vi "Ex6.vi"() -> ()   [LabVIEW 2016]
uses:
  <vilib>/DAQmx/create/channels.llb/DAQmx Create Channel (CO-Pulse Generation-Frequency).vi
  <vilib>/DAQmx/configure/timing.llb/DAQmx Timing (Implicit).vi
  <vilib>/DAQmx/miscellaneous.llb/DAQmx Fill In Error Info.vi
  <vilib>/DAQmx/create/channels.llb/DAQmx Create Channel (CI-Period).vi
  <vilib>/DAQmx/read.llb/DAQmx Read (Counter DBL 1Chan 1Samp).vi
panel:
  in  "frequency":dbl=1.0 caption="주파수" format="%.6f"
  in  "counter 2":tag caption="카운터"
  out "data":dbl caption="주기" format="%.8p"
  in  "counter":tag caption="카운터"
  in  "정지":bool
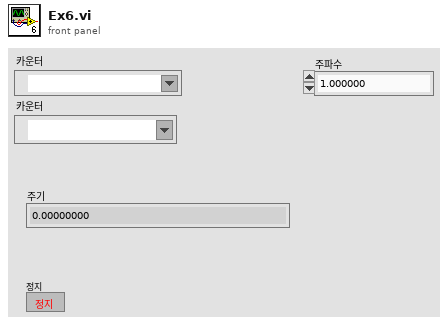
[diagram p1: front panel]
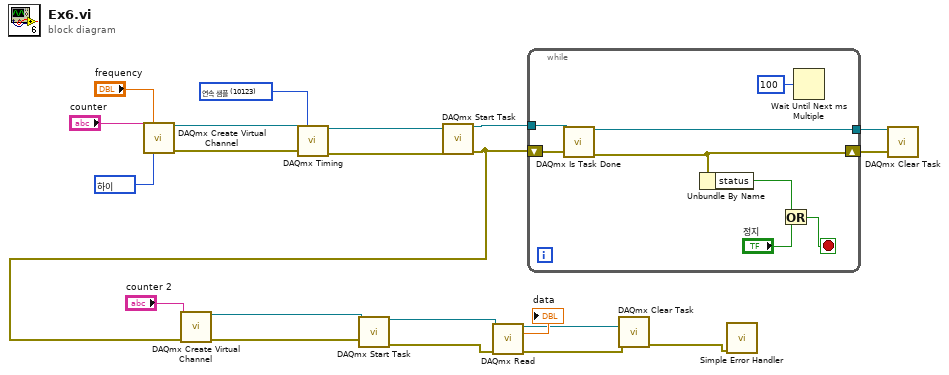
[diagram p0: block diagram]
diagram:
  w1 = 10192 items=["하이"=10192, "로우"=10214] ("idle state")
  w13 = 10123 items=["유한 샘플"=10178, "연속 샘플"=10123, "하드웨어 타이밍에 의한 단일 포인트"=12522] ("sample mode")
  n1 = call-poly <vilib>:"DAQmx Create Virtual Channel.vi"("frequency"="frequency", "counter"="counter", "idle state"=w1) -> ("task out"=w21:refnum<k21>, "error out"=w20:errorcluster)  [unwired: 11 in]
  n2 = call-poly <vilib>:"DAQmx Timing.vi"("task/channels in"=w21, "sample mode"=w13, "error in"=w20) -> ("task out"=w16:refnum<k21>, "error out"=w15:errorcluster)  [unwired: 11 in]
  n3 = call <vilib>:"DAQmx Start Task.vi"("task/channels in"=w16, "error in"=w15) -> ("task out"=w14:refnum<k21>, "error out"=w4:errorcluster)  [unwired: 12 in]
  n4 = call-poly <vilib>:"DAQmx Create Virtual Channel.vi"("counter"="counter 2", "error in"=w4) -> ("task out"=w12:refnum<k21>, "error out"=w11:errorcluster)  [unwired: 12 in]
  n5 = call <vilib>:"DAQmx Start Task.vi"("task/channels in"=w12, "error in"=w11) -> ("task out"=w10:refnum<k21>, "error out"=w9:errorcluster)  [unwired: 12 in]
  n6 = call-poly <vilib>:"DAQmx Read.vi"("task/channels in"=w10, "error in"=w9) -> ("task out"=w7:refnum<k21>, "data"=→"data":dbl, "error out"=w6:errorcluster)  [unwired: 11 in]
  n7 = while {
    shift-right: [w27] -> w19
    shift-left: w4 -> [w29]
    tunnel: [w28] -> w18
    tunnel: w14 -> [w23]
    stop <- w24 stop-if-true
    n8 = call <vilib>:"DAQmx Is Task Done.vi"("task/channels in"=w23, "error in"=w29) -> ("task out"=w28:refnum<k21>, "error out"=w27:errorcluster)  [unwired: 11 in, 1 out]
    n9 = Unbundle By Name(w27) -> ("status"=w26:bool)
    n10 = Or(x=w26, y="정지") -> (x .or. y?=w24:bool)
    n11 = Wait Until Next ms Multiple(millisecond multiple=u32 100 ("대기 시간 (ms)")) -> ()  [unwired: 1 out]
  }
  n12 = call <vilib>:"DAQmx Clear Task.vi"("task in"=w7, "error in"=w6) -> ("error out"=w5:errorcluster)  [unwired: 13 in]
  n13 = call <vilib>:"Simple Error Handler.vi"("error in (no error)"=w5) -> ()  [unwired: 4 in, 5 out]
  n14 = call <vilib>:"DAQmx Clear Task.vi"("task in"=w18, "error in"=w19) -> ()  [unwired: 13 in, 1 out]
